vi "test_Create Data Channel_single channel enumerated list.vi"(8 "error in (no error)":errorcluster, 11 "TestCase in":refnum<class "Instrument Addon Scripting API Channels Unit Tests.lvclass">) -> (0 "error out":errorcluster, 3 "TestCase out":refnum<class "Instrument Addon Scripting API Channels Unit Tests.lvclass">)   [LabVIEW 2019, in "Instrument Addon Scripting API Channels Unit Tests.lvclass"]
uses:
  Instrument Addon Scripting API Channels Unit Tests.lvclass
  APIs/Scripting API/TypeDefs/Single Channel Enumerated List Settings.ctl
  Addon/Addon Shared/Types/Protocol Data Type.ctl
  Addon/Addon Shared/Types/Data Channel Type.ctl
  Instrument Addon Scripting API Channels Unit Tests.lvclass/Instrument Addon Scripting API Channels Unit Tests.ctl
  Addon/Addon Shared/SubVIs/Constants.vi
  <vilib>/NI/NI VeriStand Advanced SysDef API/_SubVIs/SysDef.Search.GUID.vi
  <vilib>/NI VeriStand/Custom Device API/Get Item Property (U16).vi
  <vilib>/NI/NI VeriStand Advanced SysDef API/_SubVIs/SysDef.Search.GUIDs.vi
  APIs/Scripting API/Channels/Create Data Channel - Single Channel - Enumerated List.vi
  <vilib>/NI VeriStand/Custom Device API/Get Item Property (String Array).vi
  <vilib>/addons/_JKI Toolkits/VI Tester/TestCase.llb/TestCase.lvclass
  <vilib>/NI/NI VeriStand Advanced SysDef API/SysDef API/Advanced System Definition.lvlib
  Addon/Addon Shared/Instrument Addon Shared.lvlib
  APIs/Scripting API/Instrument Addon Scripting API.lvlib
  <vilib>/NI VeriStand/Custom Device API/Custom Device API.lvlib
  C:/Program Files (x86)/National Instruments/LabVIEW 2019/vi.lib/addons/_JKI Toolkits/VI Tester/TestCase.llb/TestCase.lvclass
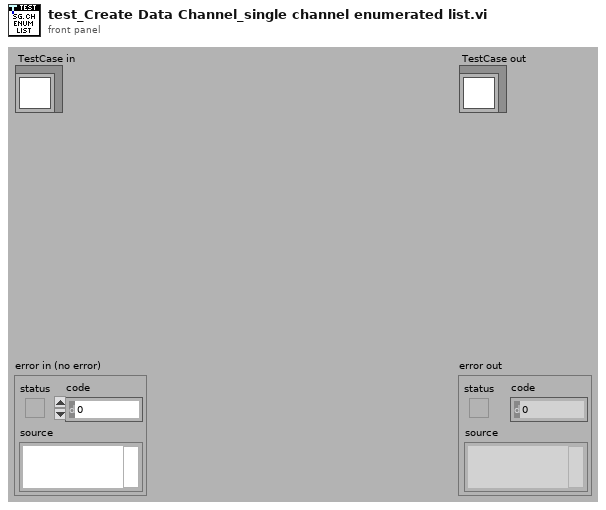
[diagram p1: front panel]
types:
  T1 = typedef "Instrument Addon Scripting API.lvlib/Single Channel Enumerated List Settings.ctl" = cluster{"Enumerated List":string[], "Default Value":dbl, "Units":string}
  T2 = typedef "Instrument Addon Shared.lvlib/Data Channel Type.ctl" = enum16{"Format", "Comparison", "Type Cast", "Enumerated List"}
  T3 = typedef "Instrument Addon Shared.lvlib/Protocol Data Type.ctl" = enum16{"Single Channel", "Array"}
  T4 = typedef "Custom Device API.lvlib/Custom Device Item Ref.ctl" = u64
  T5 = typedef "Custom Device API.lvlib/Custom Device Channel.ctl" = cluster{"Type":T6, "Units":string, "Default Value":dbl, "Faultable":bool, "Scalable":bool}
  T6 = typedef "Custom Device API.lvlib/Custom Device Channel Type.ctl" = enum16{"Input", "Output"}
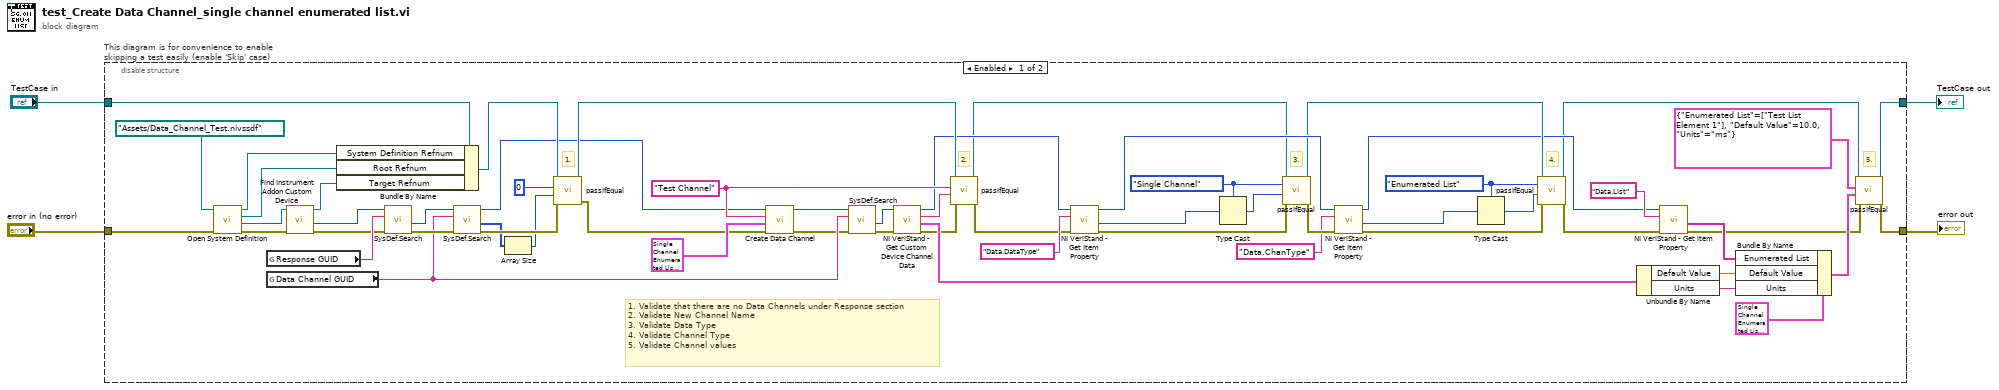
[diagram p0: block diagram]
diagram:
  n1 = disable-structure "This diagram is for convenience to enable skipping a test easily (enable 'Skip' case)" shown="Enabled" {
    disable-tunnel: "TestCase in" -> [w30 w68]
    disable-tunnel: [w64 w66] -> w1
    disable-tunnel: [w63 w67] -> w3
    disable-tunnel: "error in (no error)" -> [w59 w65]
    frame Enabled {
      w17 = Data_Channel_Type."Enumerated List" ("Channel Type")
      w22 = Protocol_Data_Type."Single Channel" ("Data Type")
      w38 = "Test Channel" ("Name")
      # "1. Validate that there are no Data Channels under Response section\n2. Validate New Channel Name\n3. Validate Data Type\n4. Validate Channel Type\n5. Validate Channel values"
      # "4."
      # "3."
      # "5."
      # "2."
      # "1."
      n2 = call "Open System Definition.vi"("error in (no error)"=w59, "System Definition File"=path "Assets/Data_Channel_Test.nivssdf") -> ("error out"=w62:errorcluster, "Target Refnum"=w61:refnum<k24>, "Root Refnum"=w33:refnum<k24>, "System Definition Refnum"=w34:refnum<k24>)  [unwired: 6 in]
      n3 = global read "Constants.vi" "Response GUID"() -> (w57:string)
      n4 = global read "Constants.vi" "Data Channel GUID"() -> (w54:string)
      n5 = call "Find Instrument Addon Custom Device.vi"("error in"=w62, "target in"=w61) -> ("error out"=w31:errorcluster, "NodeID"=w58:u64, "target out"=w32:refnum<k24>)  [unwired: 7 in]
      n6 = Bundle By Name(cluster=w30, "System Definition Refnum"=w34, "Root Refnum"=w33, "Target Refnum"=w32) -> (w29:refnum<class "Instrument Addon Scripting API Channels Unit Tests.lvclass">)
      n7 = call-poly <vilib>:"SysDef.Search.vi"("error in (no error)"=w31, "GUID"=w57, "nodeID"=w58) -> ("error out"=w55:errorcluster, "Value out"=w56:u64)  [unwired: 5 in, 2 out]
      n8 = call-poly <vilib>:"SysDef.Search.vi"("error in (no error)"=w55, "GUID"=w54, "nodeID"=w56) -> ("error out"=w43:errorcluster, "Values Out"=w42:u64[], "nodeID out"=w5:u64)  [unwired: 5 in, 1 out]
      n9 = Array Size(array=w42) -> (size(s)=w41:i32)
      n10 = call-dynamic "passIfEqual.vi"("error in (no error)"=w43, "y"=w41, "x"=0 ("size(s)"), "TestCase in"=w29) -> ("error out"=w28:errorcluster, "TestCase out"=w27:refnum<class "Instrument Addon Scripting API Channels Unit Tests.lvclass">)  [unwired: 6 in]
      n11 = call-poly "Create Data Channel.vi"("error in (no error)"=w28, "settings"=T1 {"Enumerated List"=["Test List Element 1"], "Default Value"=10.0, "Units"="ms"} ("Settings"), "channel name"=w38, "response refnum in"=w5) -> ("error out"=w35:errorcluster, "response refnum out"=w36:T4)  [unwired: 5 in, 1 out]
      n12 = call-poly <vilib>:"SysDef.Search.vi"("error in (no error)"=w35, "GUID"=w54, "nodeID"=w36) -> ("error out"=w53:errorcluster, "Value out"=w52:u64)  [unwired: 5 in, 2 out]
      n13 = call <vilib>:"NI VeriStand - Get Custom Device Channel Data.vi"("error in (no error)"=w53, "Channel Ref in"=w52) -> ("error out"=w12:errorcluster, "Channel"=w49:T5, "Channel Name"=w45:string, "Channel Ref out"=w13:T4)  [unwired: 4 in, 2 out]
      n14 = call-dynamic "passIfEqual.vi"("error in (no error)"=w12, "y"=w45, "x"=w38, "TestCase in"=w27) -> ("error out"=w11:errorcluster, "TestCase out"=w10:refnum<class "Instrument Addon Scripting API Channels Unit Tests.lvclass">)  [unwired: 6 in]
      n15 = call-poly <vilib>:"NI VeriStand - Get Item Property.vi"("error in (no error)"=w11, "Property Name"="Data.DataType", "Item Ref in"=w13) -> ("error out"=w25:errorcluster, "Value"=w24:u16, "Item Ref out"=w16:T4)  [unwired: 5 in, 1 out]
      n16 = Type Cast(type=w22, x=w24) -> (*(type *) &x=w23:T3)
      n17 = call-dynamic "passIfEqual.vi"("error in (no error)"=w25, "y"=w23, "x"=w22, "TestCase in"=w10) -> ("error out"=w21:errorcluster, "TestCase out"=w14:refnum<class "Instrument Addon Scripting API Channels Unit Tests.lvclass">)  [unwired: 6 in]
      n18 = call-poly <vilib>:"NI VeriStand - Get Item Property.vi"("error in (no error)"=w21, "Property Name"="Data.ChanType", "Item Ref in"=w16) -> ("error out"=w20:errorcluster, "Value"=w19:u16, "Item Ref out"=w8:T4)  [unwired: 5 in, 1 out]
      n19 = Type Cast(type=w17, x=w19) -> (*(type *) &x=w18:T2)
      n20 = call-dynamic "passIfEqual.vi"("error in (no error)"=w20, "y"=w18, "x"=w17, "TestCase in"=w14) -> ("error out"=w9:errorcluster, "TestCase out"=w7:refnum<class "Instrument Addon Scripting API Channels Unit Tests.lvclass">)  [unwired: 6 in]
      n21 = Unbundle By Name(w49) -> ("Default Value"=w48:dbl, "Units"=w47:string)
      n22 = call-poly <vilib>:"NI VeriStand - Get Item Property.vi"("error in (no error)"=w9, "Property Name"="Data.List", "Item Ref in"=w8) -> ("error out"=w6:errorcluster, "Value"=w50:string[])  [unwired: 5 in, 2 out]
      n23 = Bundle By Name(cluster=T1 {"Enumerated List"=["Test List Element 1"], "Default Value"=10.0, "Units"="ms"} ("Settings"), "Enumerated List"=w50, "Default Value"=w48, "Units"=w47) -> (w44:T1)
      n24 = call-dynamic "passIfEqual.vi"("error in (no error)"=w6, "y"=w44, "x"=T1 {"Enumerated List"=["Test List Element 1"], "Default Value"=10.0, "Units"="ms"} ("Settings"), "TestCase in"=w7) -> ("error out"=w63:errorcluster, "TestCase out"=w64:refnum<class "Instrument Addon Scripting API Channels Unit Tests.lvclass">)  [unwired: 6 in]
    }
    frame Disabled {
      # "skip test result while test is under development"
      n25 = call <vilib>:"skip.vi"("error in (no error)"=w65, "TestCase in"=w68) -> ("error out"=w67:errorcluster, "TestCase out"=w66:refnum<class "Instrument Addon Scripting API Channels Unit Tests.lvclass">)  [unwired: 8 in]
    }
  }
  "error out" <- w3
  "TestCase out" <- w1
